vi "Write Shape.vi"(8 "error in (no error)":errorcluster, 10 "Shape":refnum<class "Shapeable.lvclass">, 11 "DrawComponent in":refnum<class "DrawComponent.lvclass">) -> (0 "error out":errorcluster, 3 "DrawComponent out":refnum<class "DrawComponent.lvclass">)   [LabVIEW 2022 SP3, in "DrawComponent.lvclass"]
uses:
  DrawComponent.lvclass
  DrawComponent.lvclass/DrawComponent.ctl
  Shapes/Shapeable/Shapeable.lvclass
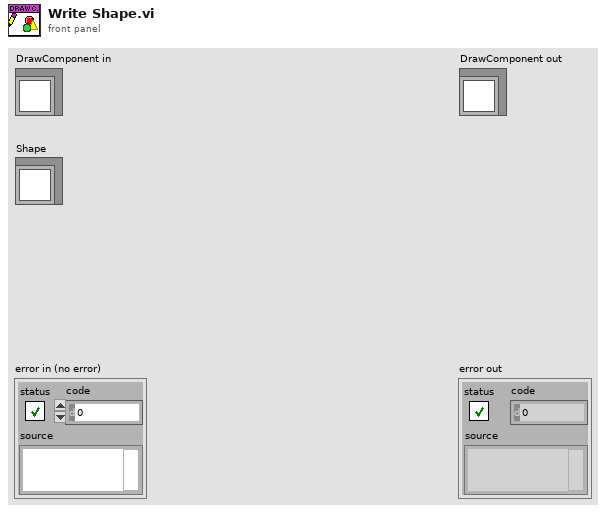
[diagram p1: front panel]
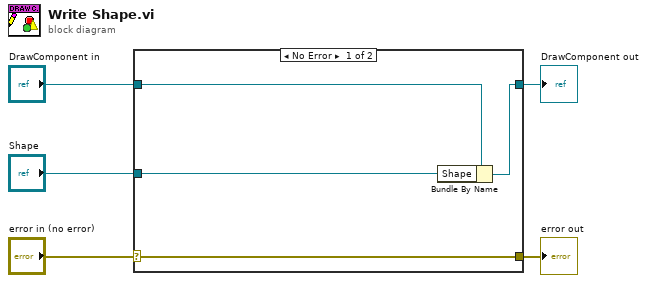
[diagram p0: block diagram]
diagram:
  n1 = case shown="No Error" "error in (no error)" {
    selector: "error in (no error)" -> [w9 w10]
    tunnel: [w9 w10] -> w4
    tunnel: [w7 w11] -> w2
    tunnel: "DrawComponent in" -> [w8 w11]
    tunnel: "Shape" -> [w6 _]
    frame No Error {
      n2 = Bundle By Name(cluster=w8, "Shape"=w6) -> (w7:refnum<class "DrawComponent.lvclass">)
    }
    frame Error {
    }
  }
  "error out" <- w4
  "DrawComponent out" <- w2
